vi "Motors_Encoders_Sensors_with_default_FPGA.vi"() -> ()   [LabVIEW 2018]
uses:
  <vilib>/myRIO/Instrument Drivers/Onboard IO/DIO/typedefs/DIO Reference.ctl
  <vilib>/myRIO/Common/Instrument Driver Framework/Utilities/typedefs/myRIO Generic Hardware Reference.ctl
  <vilib>/myRIO/Common/Instrument Driver Framework/Utilities/typedefs/Hardware Version Enum.ctl
  <vilib>/myRIO/Common/Instrument Driver Framework/Utilities/typedefs/myRIO v1.0 Reference.ctl
  <vilib>/myRIO/Common/Instrument Driver Framework/Utilities/typedefs/Generic FPGA Reference.ctl
  <vilib>/myRIO/Common/Instrument Driver Framework/myRIO v1.0/DIO/typedefs/DIO Channels List.ctl
  <vilib>/myRIO/Common/Instrument Driver Framework/myRIO v1.0/DIO/typedefs/DIO Channels Enum.ctl
  <vilib>/userdefined/High Color/nirio_resource_hc.ctl
  <vilib>/myRIO/Instrument Drivers/Onboard IO/PWM/typedefs/PWM Reference.ctl
  <vilib>/myRIO/Common/Instrument Driver Framework/myRIO v1.0/PWM/typedefs/PWM Channels Enum.ctl
  <vilib>/myRIO/Instrument Drivers/Onboard IO/PWM/typedefs/PWM Configuration.ctl
  <vilib>/myRIO/Instrument Drivers/Onboard IO/AI/typedefs/AI Reference.ctl
  <vilib>/myRIO/Common/Instrument Driver Framework/myRIO v1.0/AI/typedefs/AI Channels List.ctl
  <vilib>/myRIO/Common/Instrument Driver Framework/myRIO v1.0/AI/typedefs/AI Channels Enum.ctl
  <vilib>/myRIO/Common/Instrument Driver Framework/Utilities/typedefs/Analog Scaling Constants List.ctl
  <vilib>/myRIO/Common/Instrument Driver Framework/Utilities/typedefs/Analog Scaling Constants.ctl
  <vilib>/myRIO/Common/Instrument Driver Framework/myRIO v1.0/Encoder/typedefs/Encoder Signal Mode.ctl
  <vilib>/myRIO/Instrument Drivers/Onboard IO/Encoder/typedefs/Encoder Reference.ctl
  <vilib>/myRIO/Common/Instrument Driver Framework/myRIO v1.0/Encoder/typedefs/Encoder Channels Enum.ctl
  <vilib>/myRIO/Common/Instrument Driver Framework/myRIO v1.0/Encoder/typedefs/Encoder Configuration v1.0.ctl
  <vilib>/myRIO/Common/Instrument Driver Framework/Utilities/vis/Is FPGA Ref Available.vi
  <vilib>/myRIO/Common/Instrument Driver Framework/myRIO v1.0/DIO/vis/myRIO v1.1 Open DIO.vi
  <vilib>/myRIO/Instrument Drivers/Onboard IO/DIO/vis/Write.vi
  <vilib>/myRIO/Common/Instrument Driver Framework/myRIO v1.0/PWM/vis/myRIO v1.1 Open PWM.vi
  <vilib>/myRIO/Instrument Drivers/Onboard IO/PWM/vis/Set Duty Cycle and Frequency.vi
  <vilib>/myRIO/Common/Instrument Driver Framework/myRIO v1.0/AI/vis/myRIO v1.1 Open AI.vi
  <vilib>/myRIO/Instrument Drivers/Onboard IO/AI/vis/Read.vi
  <vilib>/myRIO/Common/Instrument Driver Framework/myRIO v1.0/Encoder/vis/myRIO v1.1 Open Encoder.vi
  <vilib>/myRIO/Instrument Drivers/Onboard IO/Encoder/vis/Read.vi
  <vilib>/myRIO/Common/Instrument Driver Framework/Utilities/vis/Validate Channels.vi
  <vilib>/myRIO/Common/Instrument Driver Framework/myRIO v1.0/DIO/vis/myRIO v1.0 Reserve DIO.vi
  <vilib>/myRIO/Common/Instrument Driver Framework/myRIO v1.0/PWM/vis/myRIO v1.0 Reserve PWM.vi
  <vilib>/myRIO/Common/Instrument Driver Framework/myRIO v1.0/AI/vis/myRIO v1.0 Reserve AI.vi
  <vilib>/myRIO/Common/Instrument Driver Framework/myRIO v1.0/Encoder/vis/myRIO v1.0 Reserve Encoder.vi
  <vilib>/myRIO/Common/Instrument Driver Framework/myRIO v1.0/Resource Manager/vis/myRIO v1.0 Reserve Channel List.vi
  <vilib>/myRIO/Common/Instrument Driver Framework/myRIO v1.0/DIO/vis/myRIO v1.0 Build MUX Configuration DIO.vi
  <vilib>/myRIO/Common/Instrument Driver Framework/myRIO v1.0/PWM/vis/myRIO v1.0 Build MUX Configuration PWM.vi
  <vilib>/myRIO/Common/Instrument Driver Framework/myRIO v1.0/AI/vis/myRIO v1.0 Build MUX Configuration AI.vi
  <vilib>/myRIO/Common/Instrument Driver Framework/myRIO v1.0/Encoder/vis/myRIO v1.0 Build MUX Configuration Encoder.vi
  <vilib>/myRIO/Common/Instrument Driver Framework/myRIO v1.0/Resource Manager/vis/myRIO v1.0 Reserve Channel.vi
  <vilib>/myRIO/Common/Instrument Driver Framework/myRIO v1.0/Resource Manager/vis/myRIO v1.0 Unreserve Channel.vi
  <vilib>/myRIO/Common/Instrument Driver Framework/myRIO v1.0/Resource Manager/vis/myRIO v1.0 Create Configuration List.vi
  <vilib>/myRIO/Common/Instrument Driver Framework/myRIO v1.0/Resource Manager/vis/myRIO v1.0 Build Mutex Name.vi
  <vilib>/Utility/VariantDataType/GetNumericInfo.vi
  <vilib>/Utility/error.llb/Error Cluster From Error Code.vi
  <vilib>/myRIO/Common/Instrument Driver Framework/myRIO v1.0/myRIO v1.1 Open.vi
  <vilib>/myRIO/Common/Instrument Driver Framework/Utilities/vis/IO Manager.vi
  <vilib>/myRIO/Common/Instrument Driver Framework/Utilities/vis/Configuration Manager.vi
  <vilib>/myRIO/Common/Instrument Driver Framework/myRIO v1.0/Resource Manager/vis/myRIO v1.0 Configure IO.vi
  <vilib>/myRIO/Common/Instrument Driver Framework/myRIO v1.0/myRIO v1.0 Close.vi
  <vilib>/myRIO/Common/Instrument Driver Framework/myRIO v1.0/DIO/vis/myRIO v1.0 Write DIO.vi
  <vilib>/myRIO/Common/Instrument Driver Framework/myRIO v1.0/PWM/vis/myRIO v1.0 Write PWM.vi
  <vilib>/myRIO/Common/Instrument Driver Framework/myRIO v1.0/AI/vis/myRIO v1.0 Get Scaling Constants AI.vi
  <vilib>/myRIO/Common/Instrument Driver Framework/myRIO v1.0/AI/vis/myRIO v1.0 Read AI.vi
  <vilib>/myRIO/Common/Instrument Driver Framework/myRIO v1.0/Encoder/vis/myRIO v1.0 Configure Encoder.vi
  <vilib>/myRIO/Common/Instrument Driver Framework/myRIO v1.0/Encoder/vis/myRIO v1.0 Read Encoder.vi
  <vilib>/myRIO/Express VI/Onboard IO/DO/DO Express VI.xnode
  <vilib>/myRIO/Instrument Drivers/Onboard IO/DIO/vis/myRIO DIO Open.xnode
  <vilib>/myRIO/Express VI/Onboard IO/PWM/PWM Express VI.xnode
  <vilib>/myRIO/Instrument Drivers/Onboard IO/PWM/vis/myRIO PWM Open.xnode
  <vilib>/myRIO/Express VI/Onboard IO/AI/AI Express VI.xnode
  <vilib>/myRIO/Instrument Drivers/Onboard IO/AI/vis/myRIO AI Open.xnode
  <vilib>/myRIO/Express VI/Onboard IO/Encoder/Encoder Express VI.xnode
  <vilib>/myRIO/Instrument Drivers/Onboard IO/Encoder/vis/myRIO Encoder Open.xnode
  <vilib>/myRIO/Common/Instrument Driver Framework/myRIO v1.0/Encoder/typedefs/Encoder Count Direction Enum.ctl
  <vilib>/myRIO/Instrument Drivers/Onboard IO/Encoder/Encoder.lvlib
  <vilib>/ptbypt/NI_PtbyPt.lvlib
  <vilib>/myRIO/Instrument Drivers/Onboard IO/AI/AI.lvlib
  <vilib>/myRIO/Instrument Drivers/Onboard IO/PWM/PWM.lvlib
  <vilib>/myRIO/Instrument Drivers/Onboard IO/DIO/DIO.lvlib
panel:
  in  "Motor 4 speed":dbl(slide) scale=-100.0..100.0
  in  "Motor 3 speed":dbl(slide) scale=-100.0..100.0
  in  "Motor 2 speed":dbl(slide) scale=-100.0..100.0
  in  "Motor 1 speed":dbl(slide) scale=-100.0..100.0
  out "error out":errorcluster
  out "IR Range":dbl
  in  "Koffset [cm]":dbl
  in  "Kscale [cm-V]":dbl=27.5
  out "Vo [V]":dbl format="%.2f"
  out "Ping Distance (m) 2":dbl
  out "Ping Distance (m) 1":dbl
  out "Counter 4":i32
  in  "Reset Encoder 4":bool
  out "Counter 3":i32
  in  "Reset Encoder 3":bool
  out "Counter 2":i32
  in  "Reset Encoder 2":bool
  out "Counter 1":i32
  in  "Reset Encoder 1":bool
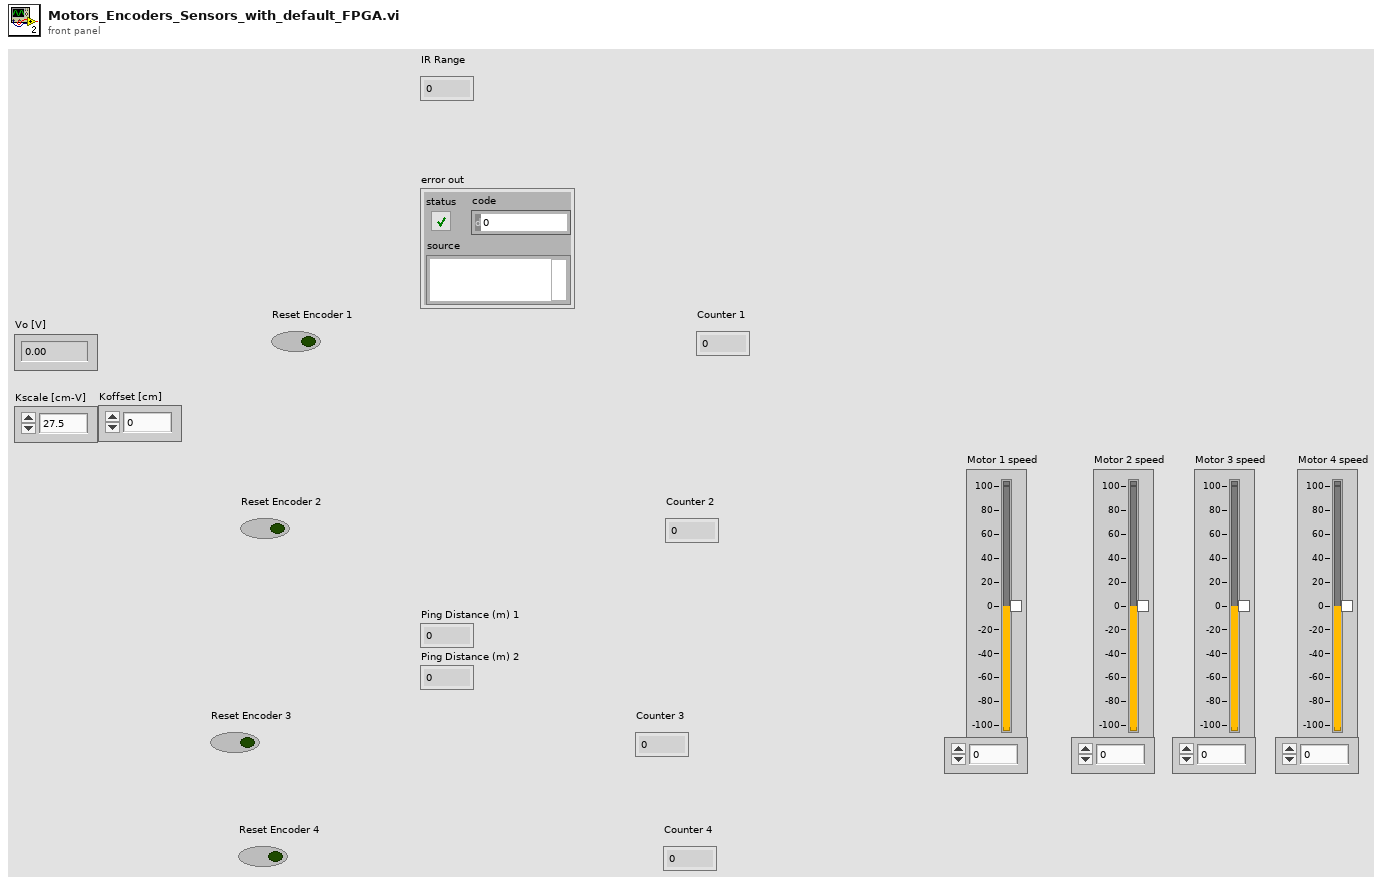
[diagram p1: front panel]
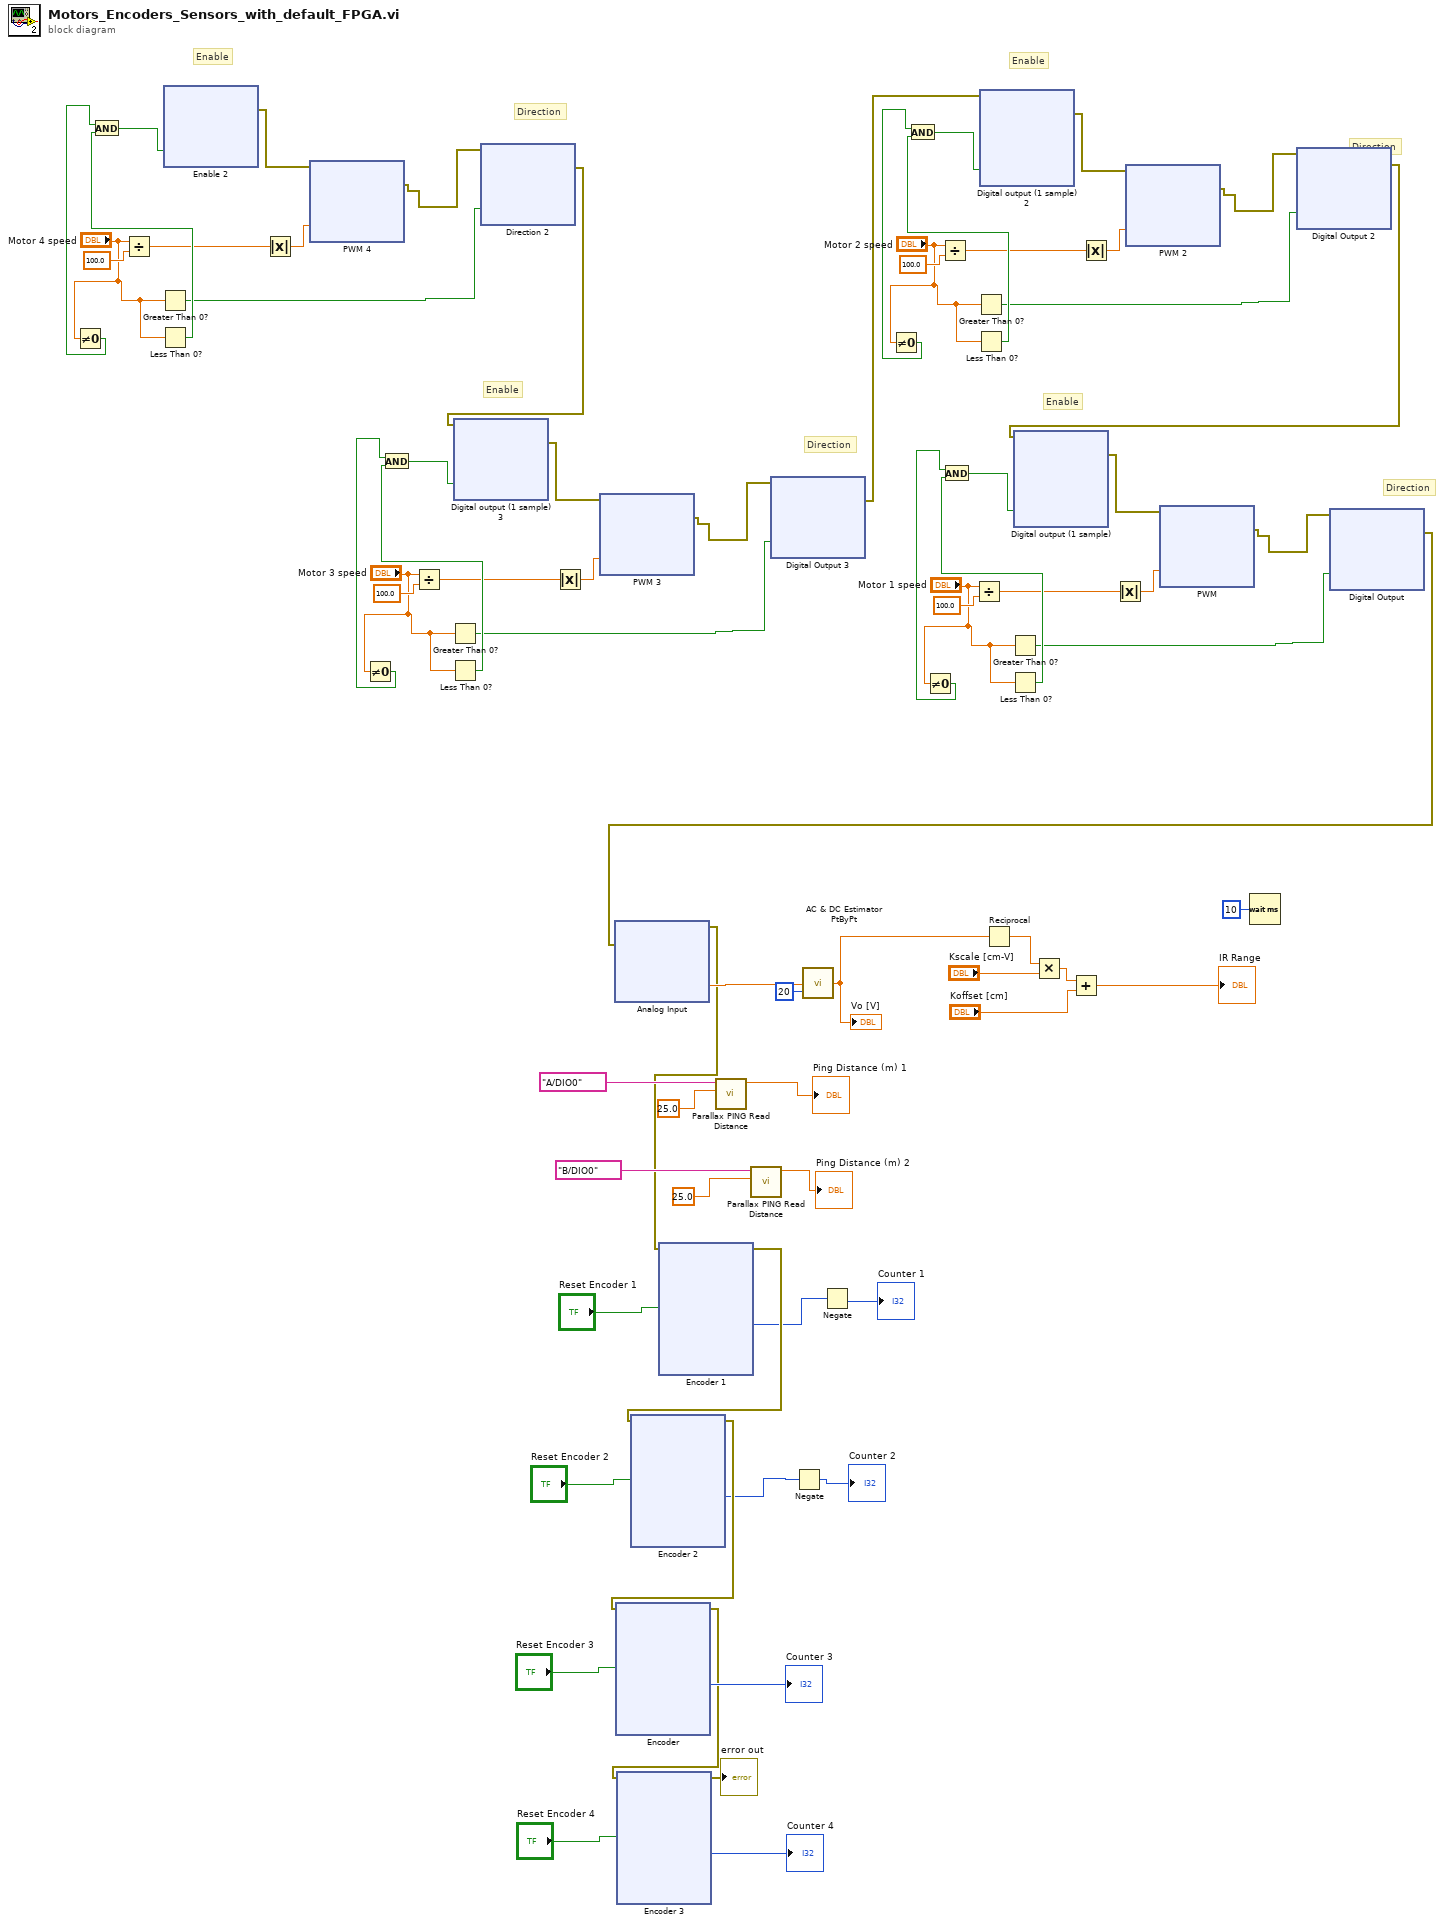
[diagram p0: block diagram]
diagram:
  # "Enable"
  # "Direction"
  # "Enable"
  # "Direction"
  # "Enable"
  # "Direction"
  # "Enable"
  # "Direction"
  n1 = Not Equal To 0?(x="Motor 4 speed") -> (x != 0?=w11:bool)
  n2 = Divide(x="Motor 4 speed", y=100.0) -> (x/y=w10:dbl)
  n3 = Greater Than 0?(x="Motor 4 speed") -> (x > 0?=w7:bool)
  n4 = Less Than 0?(x="Motor 4 speed") -> (x < 0?=w13:bool)
  n5 = And(x=w11, y=w13) -> (x .and. y?=w6:bool)
  n6 = xnode "Enable 2"("B/DIO7 (Pin 25)"=w6) -> ("error out"=w14:errorcluster)  [unwired: 1 in]
  n7 = Absolute Value(x=w10) -> (abs(x)=w9:dbl)
  n8 = xnode "PWM 4"("Duty Cycle"=w9, "error in (no error)"=w14) -> ("error out"=w15:errorcluster)
  n9 = Not Equal To 0?(x="Motor 3 speed") -> (x != 0?=w23:bool)
  n10 = Divide(x="Motor 3 speed", y=100.0) -> (x/y=w22:dbl)
  n11 = Greater Than 0?(x="Motor 3 speed") -> (x > 0?=w18:bool)
  n12 = Less Than 0?(x="Motor 3 speed") -> (x < 0?=w25:bool)
  n13 = And(x=w23, y=w25) -> (x .and. y?=w17:bool)
  n14 = xnode "Direction 2"("B/DIO13 (Pin 26)"=w7, "error in (no error)"=w15) -> ("error out"=w8:errorcluster)
  n15 = xnode "Digital output (1 sample) 3"("A/DIO7 (Pin 25)"=w17, "error in (no error)"=w8) -> ("error out"=w26:errorcluster)
  n16 = Absolute Value(x=w22) -> (abs(x)=w21:dbl)
  n17 = xnode "PWM 3"("Duty Cycle"=w21, "error in (no error)"=w26) -> ("error out"=w27:errorcluster)
  n18 = call "Parallax PING Read Distance.vi"("Temperature (deg C)"=25.0, "myRIO DIO Channel"=tag "A/DIO0") -> ("Distance (m)"=→"Ping Distance (m) 1":dbl)  [unwired: 8 in, 1 out]
  n19 = call "Parallax PING Read Distance.vi"("Temperature (deg C)"=25.0, "myRIO DIO Channel"=tag "B/DIO0") -> ("Distance (m)"=→"Ping Distance (m) 2":dbl)  [unwired: 8 in, 1 out]
  n20 = xnode "Digital Output 3"("A/DIO13 (Pin 26)"=w18, "error in (no error)"=w27) -> ("error out"=w20:errorcluster)
  n21 = Not Equal To 0?(x="Motor 2 speed") -> (x != 0?=w33:bool)
  n22 = Not Equal To 0?(x="Motor 1 speed") -> (x != 0?=w43:bool)
  n23 = Divide(x="Motor 2 speed", y=100.0) -> (x/y=w32:dbl)
  n24 = Divide(x="Motor 1 speed", y=100.0) -> (x/y=w40:dbl)
  n25 = Greater Than 0?(x="Motor 2 speed") -> (x > 0?=w30:bool)
  n26 = Less Than 0?(x="Motor 2 speed") -> (x < 0?=w35:bool)
  n27 = And(x=w33, y=w35) -> (x .and. y?=w29:bool)
  n28 = xnode "Digital output (1 sample) 2"("B/DIO5 (Pin 21)"=w29, "error in (no error)"=w20) -> ("error out"=w36:errorcluster)
  n29 = Greater Than 0?(x="Motor 1 speed") -> (x > 0?=w42:bool)
  n30 = Less Than 0?(x="Motor 1 speed") -> (x < 0?=w45:bool)
  n31 = And(x=w43, y=w45) -> (x .and. y?=w41:bool)
  n32 = Absolute Value(x=w32) -> (abs(x)=w31:dbl)
  n33 = Absolute Value(x=w40) -> (abs(x)=w39:dbl)
  n34 = xnode "PWM 2"("Duty Cycle"=w31, "error in (no error)"=w36) -> ("error out"=w37:errorcluster)
  n35 = Wait (ms)(milliseconds to wait=u32 10) -> ()  [unwired: 1 out]
  n36 = xnode "Digital Output 2"("B/DIO6 (Pin 23)"=w30, "error in (no error)"=w37) -> ("error out"=w19:errorcluster)
  n37 = xnode "Digital output (1 sample)"("A/DIO5 (Pin 21)"=w41, "error in (no error)"=w19) -> ("error out"=w46:errorcluster)
  n38 = xnode "PWM"("Duty Cycle"=w39, "error in (no error)"=w46) -> ("error out"=w47:errorcluster)
  n39 = xnode "Digital Output"("A/DIO6 (Pin 23)"=w42, "error in (no error)"=w47) -> ("error out"=w5:errorcluster)
  n40 = xnode "Analog Input"("error in (no error)"=w5) -> ("A/AI0 (Pin 3)"=w60:dbl, "error out"=w53:errorcluster)
  n41 = xnode "Encoder 1"("Reset Counter"="Reset Encoder 1", "error in (no error)"=w53) -> ("Counter Value"=w1:i32, "error out"=w52:errorcluster)  [unwired: 2 out]
  n42 = xnode "Encoder 2"("Reset Counter"="Reset Encoder 2", "error in (no error)"=w52) -> ("Counter Value"=w3:i32, "error out"=w51:errorcluster)  [unwired: 2 out]
  n43 = xnode "Encoder"("Reset Counter"="Reset Encoder 3", "error in (no error)"=w51) -> ("Counter Value"=→"Counter 3":i32, "error out"=w50:errorcluster)  [unwired: 2 out]
  n44 = xnode "Encoder 3"("Reset Counter"="Reset Encoder 4", "error in (no error)"=w50) -> ("Counter Value"=→"Counter 4":i32, "error out"=→"error out":errorcluster)  [unwired: 2 out]
  n45 = Negate(x=w3) -> (-x=→"Counter 2":i32)
  n46 = call <vilib>:"AC & DC Estimator PtByPt.vi"("signal"=w60, "sample length"=20) -> ("DC estimate (V)"=w59:dbl)  [unwired: 1 in, 2 out]
  "Vo [V]" <- w59
  n47 = Negate(x=w1) -> (-x=→"Counter 1":i32)
  n48 = Reciprocal(x=w59) -> (1/x=w62:dbl)
  n49 = Multiply(x=w62, y="Kscale [cm-V]") -> (x*y=w56:dbl)
  n50 = Add(x=w56, y="Koffset [cm]") -> (x+y=→"IR Range":dbl)
